vi "Read (Single Waveform).vi"(8 "error in (no error)":errorcluster, 9 "Maximum Time (10000 ms)":u32=10000, 10 "Channel (0: Channel 1)":u16(ring) format="%#_5f" items=["Channel 1", "Channel 2", "Channel 3", "Channel 4", "Math 1", "Math 2", "Math 3", "Math 4", "Reference 1", "Reference 2", "Reference 3", "Reference 4"], 11 "VISA resource name":refnum<visa-resource-name>) -> (0 "error out":errorcluster, 2 "Waveform Data":waveform(dbl)(graph)={"t0"=timestamp(1.815305999999491e-07 s since 1904-01-01), "dt"=5e-07, "Y"=array[10000 elements]}, 3 "VISA resource name out":refnum<visa-resource-name>)   [LabVIEW 2011, in "Tektronix 7000 Series.lvlib"]
doc: "Initiates an acquisition on all channels that you enabled with the Configure Channel VI. This VI waits for the acquisition to complete and returns the waveform for the <B>Channel</B> you specify. If the oscilloscope does not complete the acquisition within the <B>Maximum Time</B> period, this VI returns a timeout error. A timeout error often occurs because the acquisition is not triggered. For example, if the trigger level is out of range of the waveform, the acquisition is not triggered.\n\nRun the Fetch Waveform VI to obtain the waveforms for each of the remaining enabled <B>Channels</B> without initiating another acquisition.\n\n<B>Note:</B> If the instrument does not support autocompensation for probe attenuation, you might need to adjust the scaling of the <B>Waveform Data</B> accordingly. You can adjust the scaling using the Configure Channel VI or manually multiplying the <B>Waveform Data</B> by the probe attenuation."
uses:
  Tektronix 7000 Series.lvlib
  Low Level/Fetch (Waveform).vi
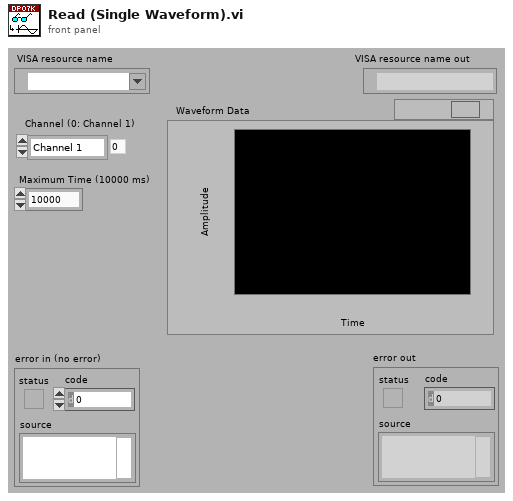
[diagram p1: front panel]
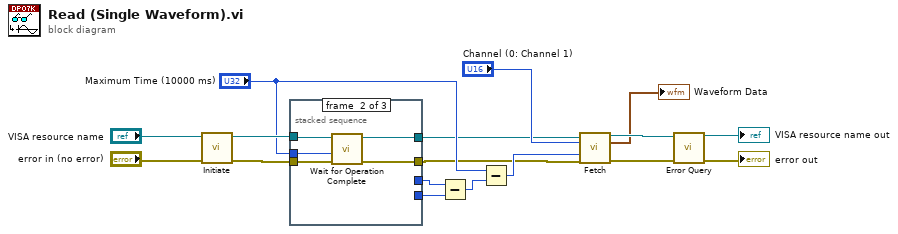
[diagram p0: block diagram]
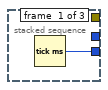
[diagram p2: hidden frame]
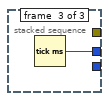
[diagram p3: hidden frame]
diagram:
  n1 = call "Initiate.vi"("error in (no error)"="error in (no error)", "VISA resource name"="VISA resource name") -> ("error out"=w5:errorcluster, "VISA resource name out"=w9:refnum<visa-resource-name>)  [unwired: 8 in]
  n2 = stacked-sequence {
    tunnel: w9 -> [_ w23 _]
    tunnel: w5 -> [_ w22 _]
    tunnel: [_ _ w24] -> w8
    tunnel: [w18 _ _] -> w7
    tunnel: "Maximum Time (10000 ms)" -> [_ w21 _]
    tunnel: [_ w20 _] -> w2
    tunnel: [_ w19 _] -> w1
    frame #0 {
      n3 = Tick Count (ms)() -> (millisecond timer value=w18:u32)
    }
    frame #1 {
      n4 = call "Wait for Operation Complete.vi"("error in (no error)"=w22, "Maximum Time (2000ms)"=w21, "VISA resource name"=w23) -> ("error out"=w19:errorcluster, "VISA resource name out"=w20:refnum<visa-resource-name>)  [unwired: 7 in]
    }
    frame #2 {
      n5 = Tick Count (ms)() -> (millisecond timer value=w24:u32)
    }
  }
  n6 = Subtract(x=w8, y=w7) -> (x-y=w6:u32)
  n7 = Subtract(x="Maximum Time (10000 ms)", y=w6) -> (x-y=w3:u32)
  n8 = call-poly "Fetch.vi"("VISA resource name"=w2, "Channel (0:Channel1)"="Channel (0: Channel 1)", "Maximum Time (10000ms)"=w3, "error in (no error)"=w1) -> ("VISA resource name out"=w15:refnum<visa-resource-name>, "Waveform Data"=→"Waveform Data":waveform(dbl), "error out"=w14:errorcluster)  [unwired: 6 in, 3 out]
  n9 = call "Error Query.vi"("error in (no error)"=w14, "VISA resource name"=w15) -> ("error out"=→"error out":errorcluster, "VISA resource name out"=→"VISA resource name out":refnum<visa-resource-name>)  [unwired: 6 in, 2 out]
